vi "通信并与其他模块交互 (子VI).vi"() -> ()   [LabVIEW 2016, in "质控单元.lvlib"]
uses:
  <vilib>/Plasmionique/MB Master/MB_Master_TCP/MB_Master_TCP.lvclass
  D:/Program Files (x86)/National Instruments/LabVIEW 2016/vi.lib/Plasmionique/MB Master/MB_Master/MB_Master.lvclass
  <vilib>/Plasmionique/MB Master/MB_Master/MB_Master.lvclass
  <vilib>/Plasmionique/MB Master/MB Master.lvlib
  <vilib>/Utility/config.llb/NI_LVConfig.lvlib
panel:
  out "队列中元素数量":i32
  out "CODCr测量状态":u16[](array[numeric])
  out "CODMn测量状态":u16[](array[numeric])
  out "总氮测量状态":u16[](array[numeric])
  out "总磷测量状态":u16[](array[numeric])
  out "氨氮测量状态":u16[](array[numeric])
  out "通讯状态":bool
  in  "starting address 6":u16
  in  "values 6":u16[](array[numeric])
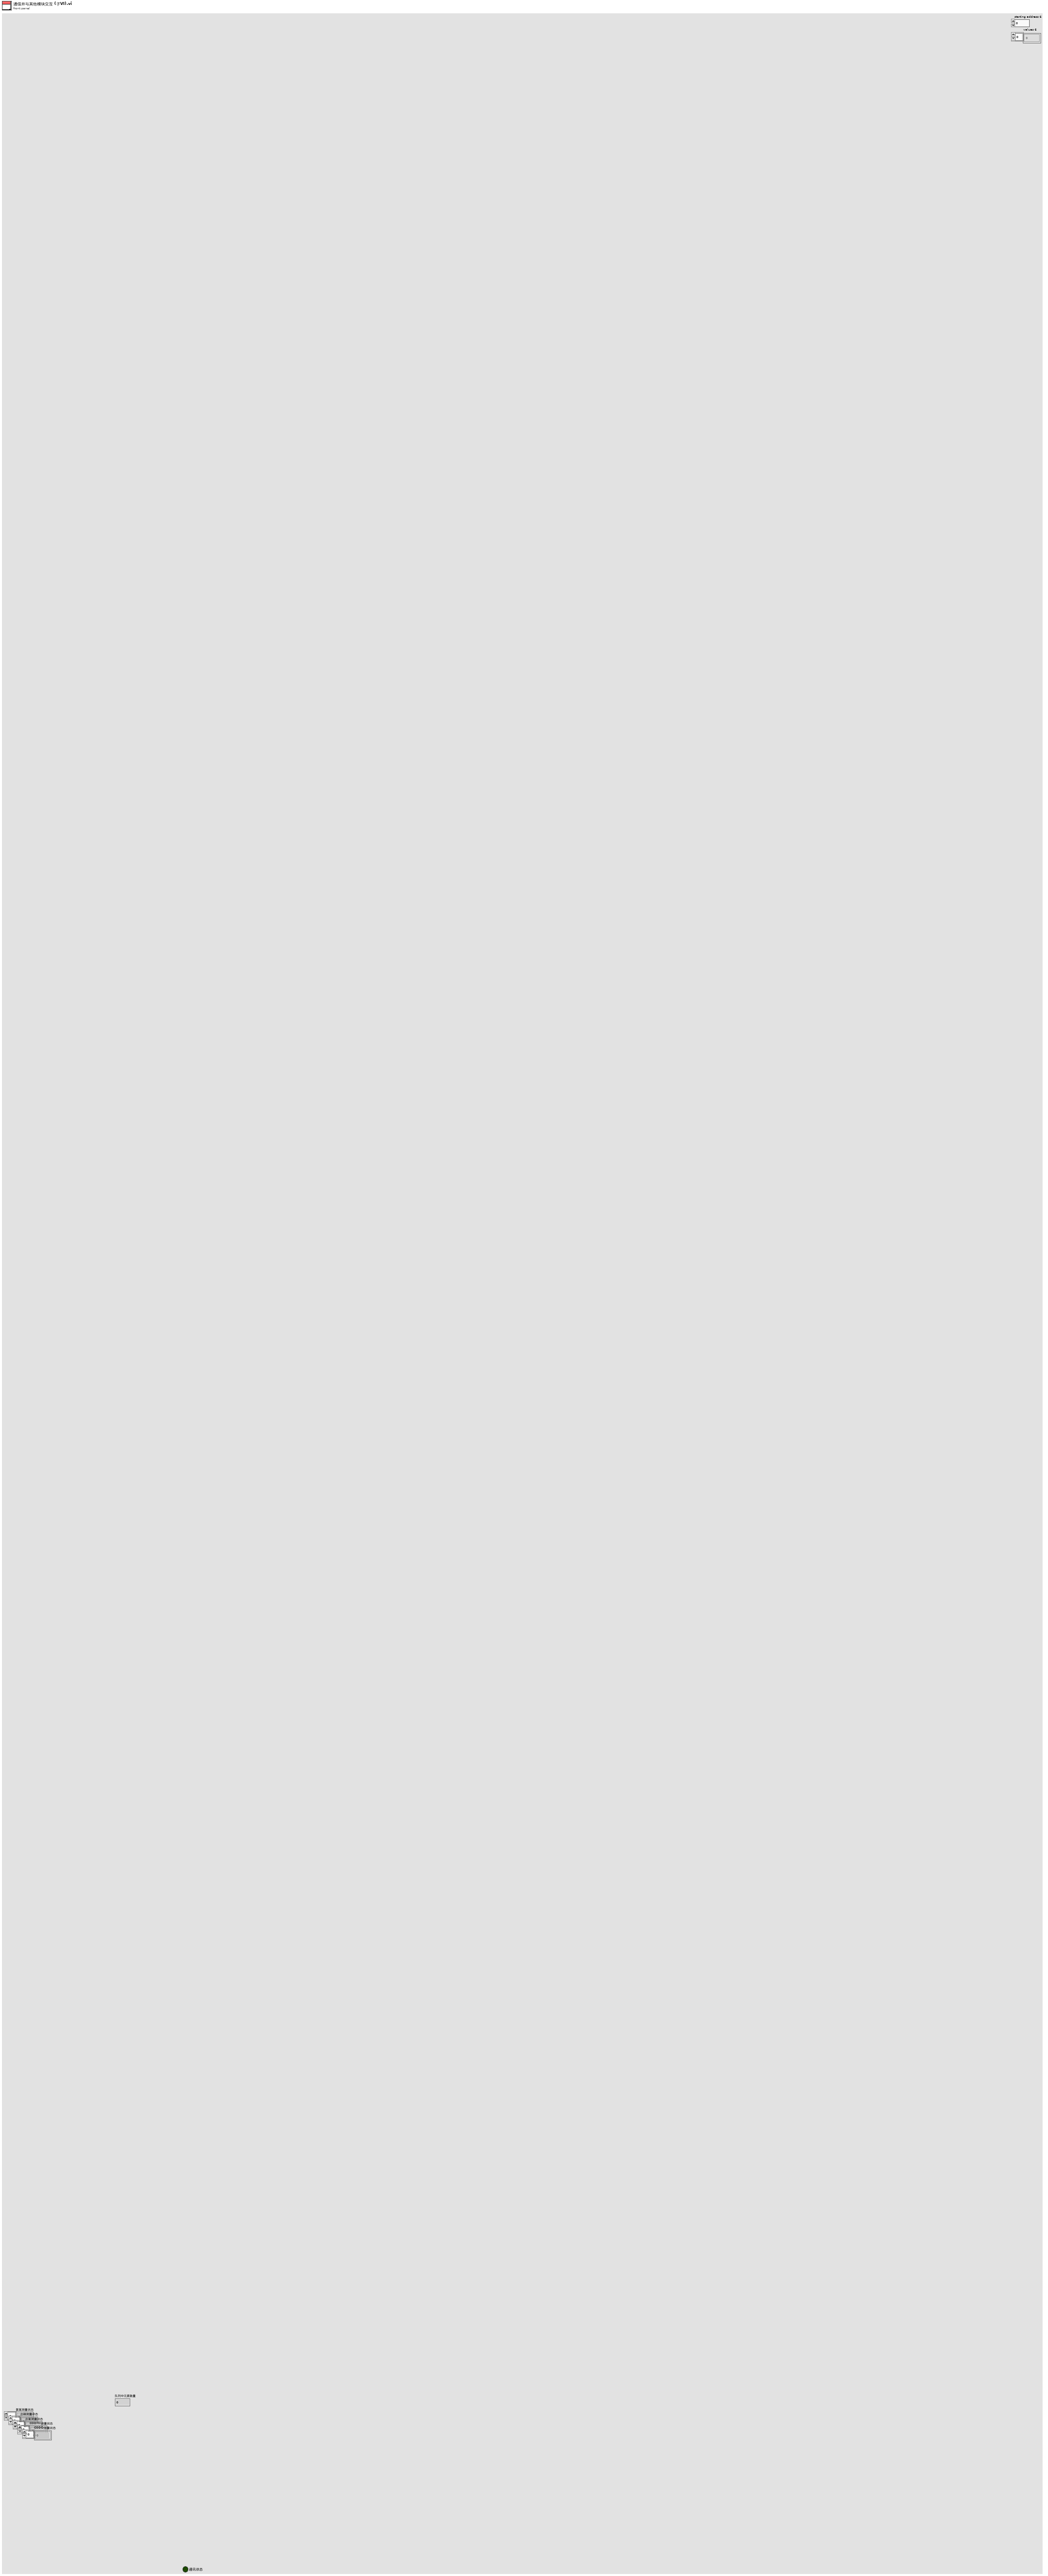
[diagram p1: front panel]
types:
  T1 = cluster{"仪器":enum16{"", "氨氮", "总磷", "总氮", "CODMn", "CODCr"}, "启动命令":enum16{"启动水样流程", "启动加标流程", "排液", "停止", "柱塞泵启动"}}
  T2 = cluster{"Registers[0]":u16, "Registers[1]":u16, "Registers[2]":u16, "Registers[3]":u16, "Registers[4]":u16, "Registers[5]":u16, "Registers[6]":u16, "Registers[7]":u16, "Registers[8]":u16, "Registers[9]":u16, "Registers[10]":u16, "Registers[11]":u16, "Registers[12]":u16, "Registers[13]":u16, "Registers[14]":u16, "Registers[15]":u16, "Registers[16]":u16, "Registers[17]":u16, "Registers[18]":u16, "Registers[19]":u16, "Registers[20]":u16, "Registers[21]":u16, "Registers[22]":u16, "Registers[23]":u16, "Registers[24]":u16, "Registers[25]":u16, "Registers[26]":u16, "Registers[27]":u16, "Registers[28]":u16, "Registers[29]":u16, "Registers[30]":u16, "Registers[31]":u16, "Registers[32]":u16, "Registers[33]":u16, "Registers[34]":u16, "Registers[35]":u16, "Registers[36]":u16, "Registers[37]":u16, "Registers[38]":u16, "Registers[39]":u16, "Registers[40]":u16, "Registers[41]":u16, "Registers[42]":u16, "Registers[43]":u16, "Registers[44]":u16, "Registers[45]":u16, "Registers[46]":u16, "Registers[47]":u16, "Registers[48]":u16, "Registers[49]":u16, "Registers[50]":u16, "Registers[51]":u16, "Registers[52]":u16, "Registers[53]":u16, "Registers[54]":u16, "Registers[55]":u16, "Registers[56]":u16}
  T3 = cluster{"因子编码":u32, "单位":u16, "标样参考值":sgl, "水样数据时间":timestamp, "水样实测值":sgl, "水样数据标识":string, "标样数据时间":timestamp, "标样实测值":sgl, "标样数据标识":string, "空白数据时间":timestamp, "空白实测值":sgl, "空白数据标识":string, "零点核查数据时间":timestamp, "零点核查实测值":sgl, "零点核查数据标识":string, "跨度核查数据时间":timestamp, "跨度核查实测值":sgl, "跨度核查数据标识":string, "加标回收数据时间":timestamp, "加标回收实测值":sgl, "加标回收数据标识":string, "平行样数据时间":timestamp, "平行样实测值":sgl, "平行样数据标识":string}
  T4 = cluster{"系统时间":timestamp, "工作状态":enum16{"空闲", "水样测试", "标样核查", "零点核查", "跨度核查", "空白测试", "平行样测试", "加标回收", "空白校准", "标样校准", "初始化（清洗）"}, "测量模式":enum16{"待机", "连续模式", "周期模式", "定点模式", "受控模式", "手动模式"}, "告警代码":enum16{"无告警", "缺试剂告警", "缺水样告警", "缺蒸馏水告警", "缺标液告警", "仪表漏液告警", "标定异常告警", "超量程告警", "加热异常", "低试剂预警", "超上限告警", "超下限告警", "仪表内部其他异常", "滴定异常告警", "电极异常告警", "量程切换告警", "参数设置告警", "PH电极电位异常", "电导率电极异常", "浊度光度异常", "溶解氧电极异常", "溶解氧光强异常", "温度异常告警", "PH异常告警", "溶解氧异常告警", "电导率异常告警", "浊度异常告警", "叶绿素异常告警", "藻密度异常告警", "蓝绿藻异常告警", "ORP异常告警", "氨氮异常告警", "清洁刷异常告警", "SD卡异常告警", "蓝牙异常告警", "Wifi异常告警", "流程异常告警"}, "故障代码":enum16{"无故障", "电机故障", "温度故障", "通讯故障", "滴定故障"}, "日志代码":u16, "软件版本":u16, "F0":sgl, "F1":sgl, "F2":sgl, "F3":sgl, "T":sgl, "H":sgl, "id":u16, "flowid":u16, "量程":u16, "总磷控温温度1":sgl, "营养盐控温温度2":sgl, "ADC":sgl}
  T5 = typedef "NI_LVConfig.lvlib/Config Data RefNum.ctl" = refnum<k1>
  T6 = cluster{"仪器":enum16{"", "氨氮", "总磷", "总氮", "CODMn", "CODCr"}, "starting address":u16, "value":u16}
  T7 = cluster{"starting address":u16, "values":u16[], "Slave ID":u8}
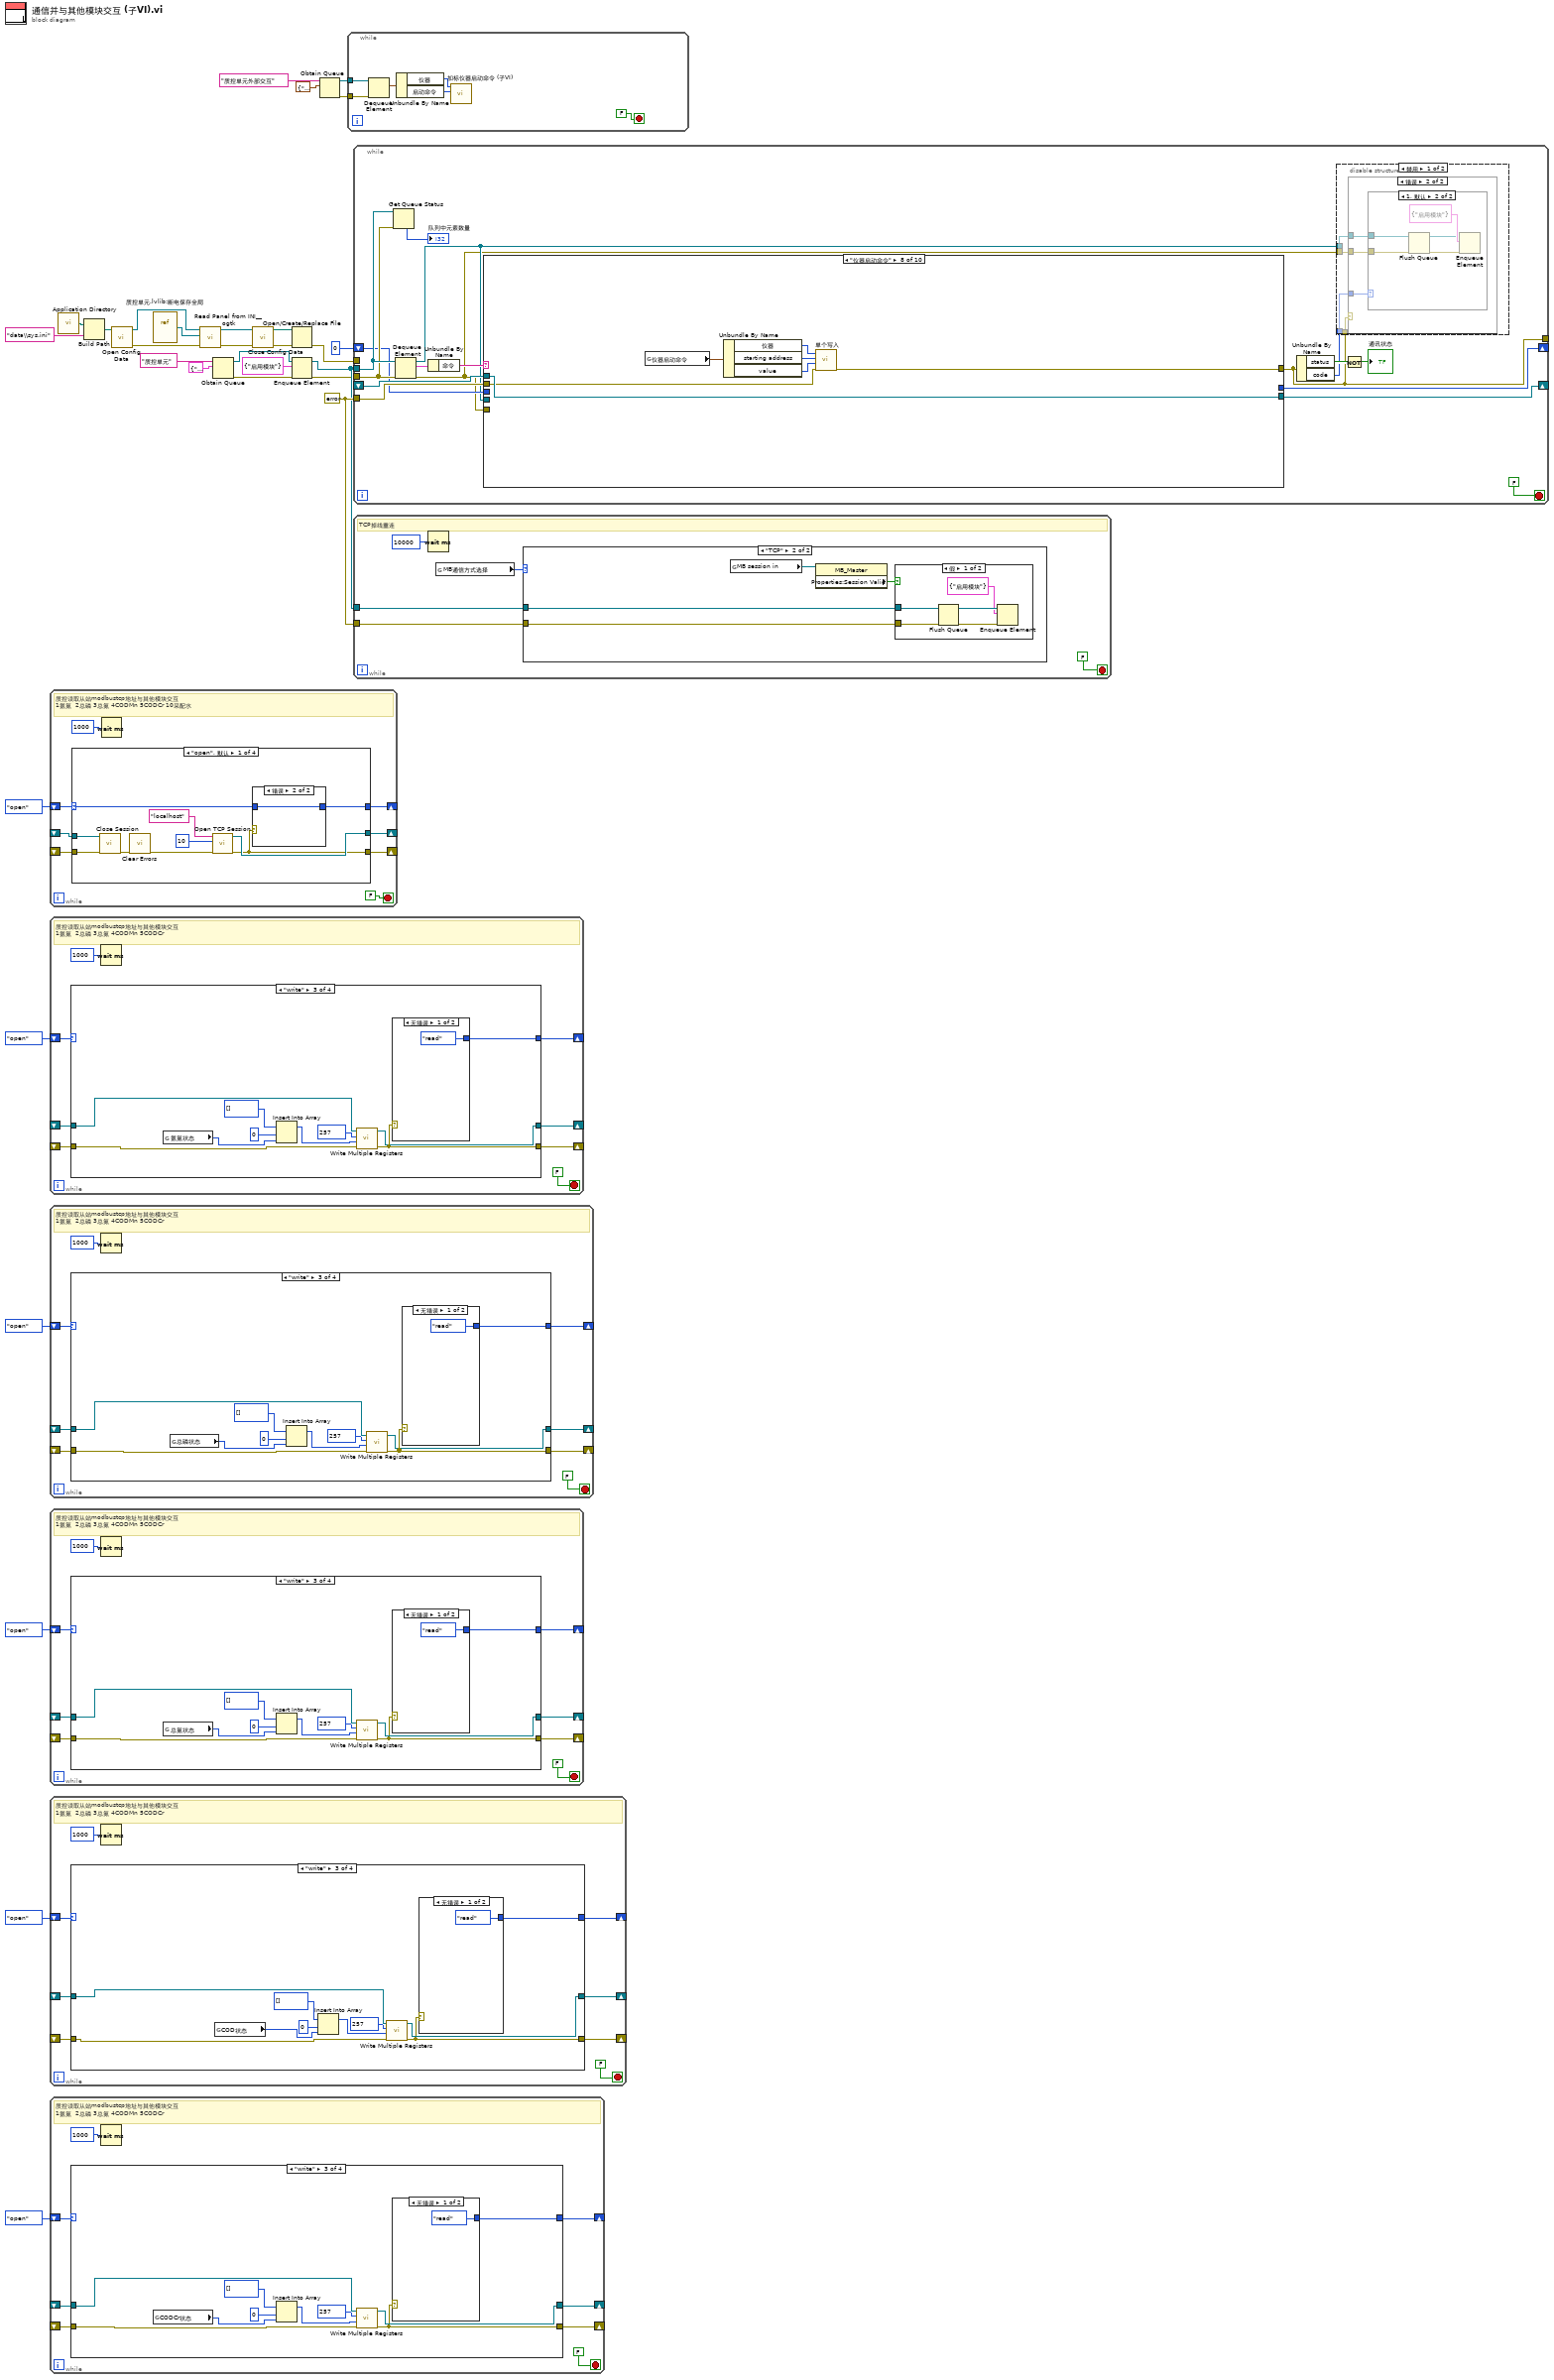
[diagram p0: block diagram]
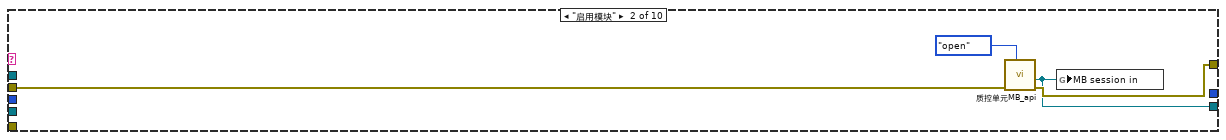
[diagram p8: hidden frame]
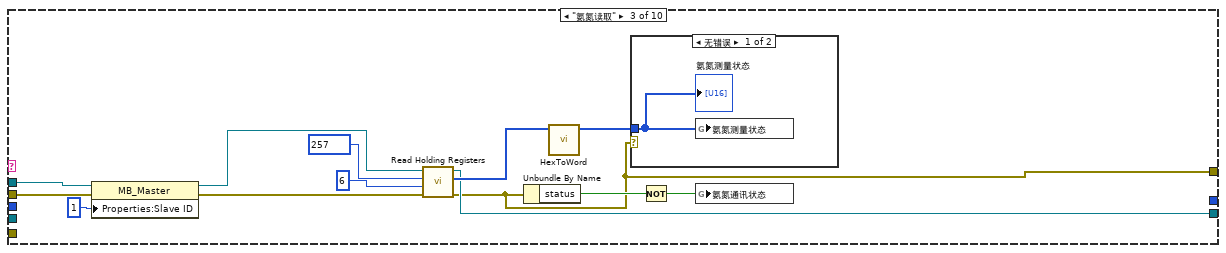
[diagram p9: hidden frame]
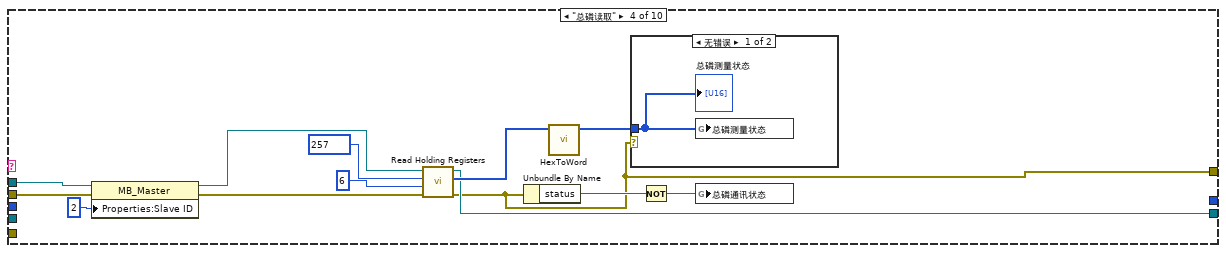
[diagram p11: hidden frame]
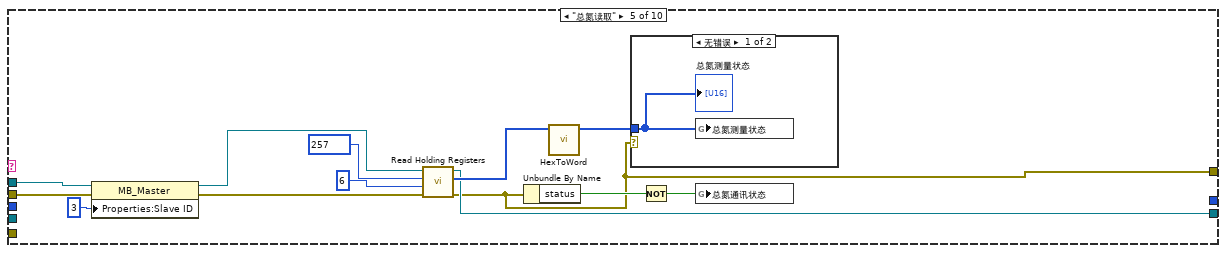
[diagram p13: hidden frame]
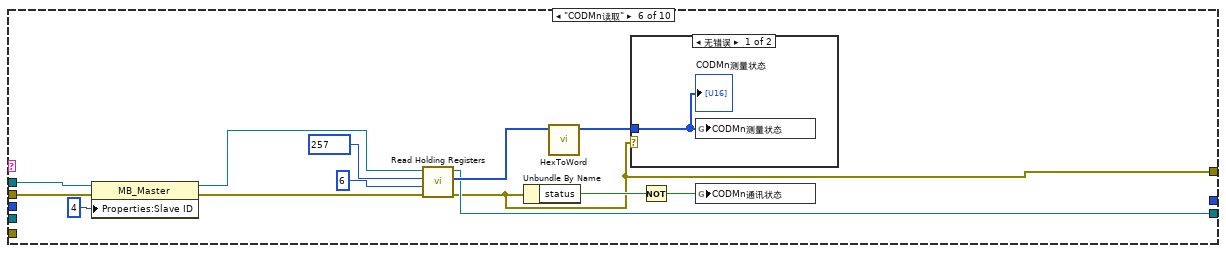
[diagram p15: hidden frame]
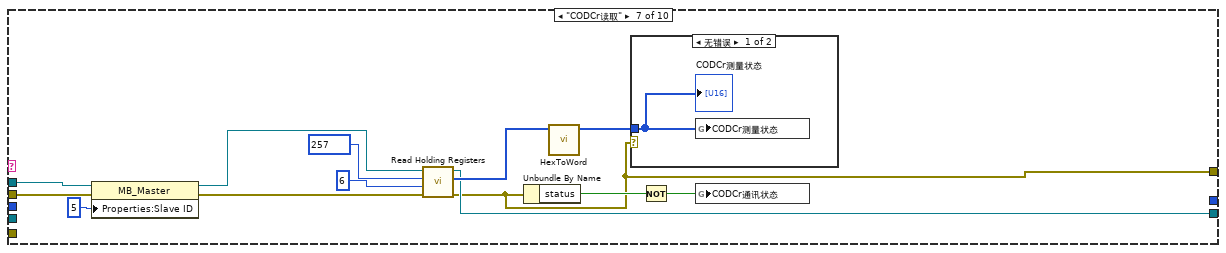
[diagram p17: hidden frame]
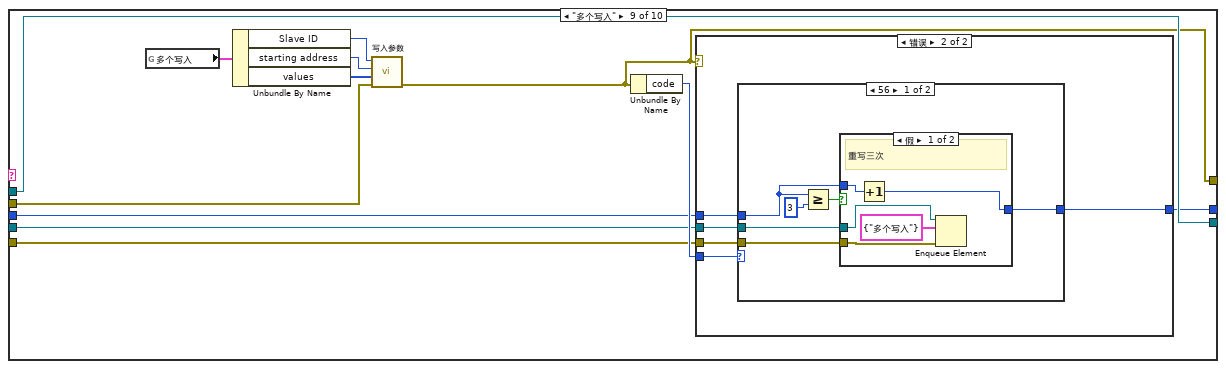
[diagram p19: hidden frame]
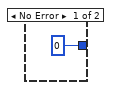
[diagram p20: hidden frame]
diagram:
  w8 = errorcluster {"status"=FALSE, "code"=0, "source"=""} ("error out")
  n1 = while {
    shift-right: [w36] -> _
    shift-left: _ -> [w38]
    shift-right: [w35] -> _
    shift-left: _ -> [w37]
    shift-right: [w32] -> _
    shift-left: enum16{"open", "read", "write", "close"}."open" -> [w33]
    stop <- FALSE stop-if-true
    # "质控读取从站modbustcp地址与其他模块交互\n1氨氮  2总磷 3总氮 4CODMn 5CODCr 10采配水"
    n2 = case shown="\"open\", 默认" w33 {
      selector: w33 -> [w40 _ _ _]
      tunnel: w38 -> [w45 w60 w68 w76]
      tunnel: w37 -> [w44 w57 w67 w75]
      tunnel: [w46 w53 w66 w76] -> w36
      tunnel: [w41 w52 w65 w73] -> w35
      tunnel: [w39 w56 w69 enum16{"open", "read", "write", "close"}."open"] -> w32
      frame "open", Default {
        n3 = call-dynamic "Close Session.vi"("error in (no error)"=w44, "MB session in"=w45) -> ("error out"=w43:errorcluster)  [unwired: 9 in]
        n4 = call <vilib>:"Clear Errors.vi"("error in (no error)"=w43) -> ("error out"=w42:errorcluster)  [unwired: 5 in, 1 out]
        n5 = call <vilib>:"Open TCP Session.vi"("error in (no error)"=w42, "Port (502)"=u16 10, "IP Address"="localhost") -> ("error out"=w41:errorcluster, "MB_TCP session"=w46:refnum<class "MB_Master_TCP.lvclass">)  [unwired: 7 in]
        n6 = case shown="错误" w41 {
          tunnel: w40 -> [w50 w51]
          tunnel: [w49 w51] -> w39
          frame No Error {
            n7 = Increment(x=w50) -> (x+1=w49:enum16{"open", "read", "write", "close"})
          }
          frame Error {
          }
        }
      }
      frame "read" {
        # "测量数据"
        n8 = call <vilib>:"Read Holding Registers.vi"("error in (no error)"=w57, "quantity"=u16 57, "starting address"=u16 0, "MB session in"=w60) -> ("error out"=w52:errorcluster, "Registers"=w55:u16[], "MB session out"=w53:refnum<class "MB_Master.lvclass">)  [unwired: 5 in]
        n9 = Array To Cluster(array=w55) -> (cluster=w54:T2)
        n10 = case shown="无错误" w52 {
          tunnel: [enum16{"open", "read", "write", "close"}."read" enum16{"open", "read", "write", "close"}."close"] -> w56
          frame No Error {
          }
          frame Error {
          }
        }
        n11 = global write "与采配水交互全局.vi" "状态"(w54) -> ()
      }
      frame "write" {
        n12 = call <vilib>:"Write Multiple Registers.vi"("error in (no error)"=w67, "values"="values 6", "starting address"="starting address 6", "MB session in"=w68) -> ("error out"=w65:errorcluster, "MB session out"=w66:refnum<class "MB_Master.lvclass">)  [unwired: 6 in]
        n13 = case shown="无错误" w65 {
          tunnel: [enum16{"open", "read", "write", "close"}."read" enum16{"open", "read", "write", "close"}."close"] -> w69
          frame No Error {
          }
          frame Error {
          }
        }
      }
      frame "close" {
        n14 = call-dynamic "Close Session.vi"("error in (no error)"=w75, "MB session in"=w76) -> ("error out"=w74:errorcluster)  [unwired: 9 in]
        n15 = call <vilib>:"Clear Errors.vi"("error in (no error)"=w74) -> ("error out"=w73:errorcluster)  [unwired: 5 in, 1 out]
      }
    }
    n16 = Wait (ms)(milliseconds to wait=u32 1000 ("等待时间（毫秒）")) -> ()  [unwired: 1 out]
  }
  n17 = while {
    shift-right: [w82] -> _
    shift-left: _ -> [w84]
    shift-right: [w81] -> _
    shift-left: _ -> [w83]
    shift-right: [w78] -> _
    shift-left: enum16{"open", "read", "write", "close"}."open" -> [w79]
    stop <- FALSE stop-if-true
    # "质控读取从站modbustcp地址与其他模块交互\n1氨氮  2总磷 3总氮 4CODMn 5CODCr"
    n18 = case shown="\"write\"" w79 {
      selector: w79 -> [w86 _ _ _]
      tunnel: w84 -> [w91 w112 w123 w131]
      tunnel: w83 -> [w90 w109 w122 w130]
      tunnel: [w92 w103 w121 w131] -> w82
      tunnel: [w87 w102 w120 w128] -> w81
      tunnel: [w85 w108 w124 enum16{"open", "read", "write", "close"}."open"] -> w78
      frame "open", Default {
        n19 = call-dynamic "Close Session.vi"("error in (no error)"=w90, "MB session in"=w91) -> ("error out"=w89:errorcluster)  [unwired: 9 in]
        n20 = call <vilib>:"Clear Errors.vi"("error in (no error)"=w89) -> ("error out"=w88:errorcluster)  [unwired: 5 in, 1 out]
        n21 = call <vilib>:"Open TCP Session.vi"("error in (no error)"=w88, "Port (502)"=u16 1, "IP Address"="localhost") -> ("error out"=w87:errorcluster, "MB_TCP session"=w92:refnum<class "MB_Master_TCP.lvclass">)  [unwired: 7 in]
        n22 = case shown="错误" w87 {
          tunnel: w86 -> [w96 w97]
          tunnel: [w95 w97] -> w85
          frame No Error {
            n23 = Increment(x=w96) -> (x+1=w95:enum16{"open", "read", "write", "close"})
          }
          frame Error {
          }
        }
      }
      frame "read" {
        # "状态告警"
        # "测量数据"
        n24 = call <vilib>:"Read Holding Registers.vi"("error in (no error)"=w109, "quantity"=u16 83, "starting address"=u16 4096, "MB session in"=w112) -> ("error out"=w104:errorcluster, "Registers"=w101:u16[], "MB session out"=w105:refnum<class "MB_Master.lvclass">)  [unwired: 5 in]
        n25 = call "交互测量数据区解析.vi"("数组"=w101) -> ("测量数据区"=w100:T3)  [unwired: 10 in]
        n26 = call <vilib>:"Read Holding Registers.vi"("error in (no error)"=w104, "quantity"=u16 24, "starting address"=u16 4224, "MB session in"=w105) -> ("error out"=w102:errorcluster, "Registers"=w99:u16[], "MB session out"=w103:refnum<class "MB_Master.lvclass">)  [unwired: 5 in]
        n27 = case shown="无错误" w102 {
          tunnel: [enum16{"open", "read", "write", "close"}."write" enum16{"open", "read", "write", "close"}."close"] -> w108
          frame No Error {
          }
          frame Error {
          }
        }
        n28 = call "交互状态告警区解析.vi"("数组"=w99) -> ("状态告警区"=w98:T4)  [unwired: 10 in]
        n29 = global write "与氨氮交互全局.vi" "氨氮测量数据区"(w100) -> ()
        n30 = global write "与氨氮交互全局.vi" "氨氮状态告警区"(w98) -> ()
      }
      frame "write" {
        n31 = global read "加标回收状态全局变量.vi" "氨氮状态"() -> (w118:u16)
        n32 = Insert Into Array(array=u16[] [] ("values 6"), index=0 ("索引"), new element=w118) -> (w115:u16[])
        n33 = call <vilib>:"Write Multiple Registers.vi"("error in (no error)"=w122, "values"=w115, "starting address"=u16 257, "MB session in"=w123) -> ("error out"=w120:errorcluster, "MB session out"=w121:refnum<class "MB_Master.lvclass">)  [unwired: 6 in]
        n34 = case shown="无错误" w120 {
          tunnel: [enum16{"open", "read", "write", "close"}."read" enum16{"open", "read", "write", "close"}."close"] -> w124
          frame No Error {
          }
          frame Error {
          }
        }
      }
      frame "close" {
        n35 = call-dynamic "Close Session.vi"("error in (no error)"=w130, "MB session in"=w131) -> ("error out"=w129:errorcluster)  [unwired: 9 in]
        n36 = call <vilib>:"Clear Errors.vi"("error in (no error)"=w129) -> ("error out"=w128:errorcluster)  [unwired: 5 in, 1 out]
      }
    }
    n37 = Wait (ms)(milliseconds to wait=u32 1000 ("等待时间（毫秒）")) -> ()  [unwired: 1 out]
  }
  n38 = while {
    shift-right: [w137] -> _
    shift-left: _ -> [w139]
    shift-right: [w136] -> _
    shift-left: _ -> [w138]
    shift-right: [w133] -> _
    shift-left: enum16{"open", "read", "write", "close"}."open" -> [w134]
    stop <- FALSE stop-if-true
    # "质控读取从站modbustcp地址与其他模块交互\n1氨氮  2总磷 3总氮 4CODMn 5CODCr"
    n39 = case shown="\"write\"" w134 {
      selector: w134 -> [w141 _ _ _]
      tunnel: w139 -> [w146 w167 w178 w186]
      tunnel: w138 -> [w145 w164 w177 w185]
      tunnel: [w147 w158 w176 w186] -> w137
      tunnel: [w142 w157 w175 w183] -> w136
      tunnel: [w140 w163 w179 enum16{"open", "read", "write", "close"}."open"] -> w133
      frame "open", Default {
        n40 = call-dynamic "Close Session.vi"("error in (no error)"=w145, "MB session in"=w146) -> ("error out"=w144:errorcluster)  [unwired: 9 in]
        n41 = call <vilib>:"Clear Errors.vi"("error in (no error)"=w144) -> ("error out"=w143:errorcluster)  [unwired: 5 in, 1 out]
        n42 = call <vilib>:"Open TCP Session.vi"("error in (no error)"=w143, "Port (502)"=u16 2, "IP Address"="localhost") -> ("error out"=w142:errorcluster, "MB_TCP session"=w147:refnum<class "MB_Master_TCP.lvclass">)  [unwired: 7 in]
        n43 = case shown="无错误" w142 {
          tunnel: w141 -> [w151 w152]
          tunnel: [w150 w152] -> w140
          frame No Error {
            n44 = Increment(x=w151) -> (x+1=w150:enum16{"open", "read", "write", "close"})
          }
          frame Error {
          }
        }
      }
      frame "read" {
        # "状态告警"
        # "测量数据"
        n45 = call <vilib>:"Read Holding Registers.vi"("error in (no error)"=w164, "quantity"=u16 83, "starting address"=u16 4096, "MB session in"=w167) -> ("error out"=w159:errorcluster, "Registers"=w156:u16[], "MB session out"=w160:refnum<class "MB_Master.lvclass">)  [unwired: 5 in]
        n46 = call "交互测量数据区解析.vi"("数组"=w156) -> ("测量数据区"=w154:T3)  [unwired: 10 in]
        n47 = call <vilib>:"Read Holding Registers.vi"("error in (no error)"=w159, "quantity"=u16 24, "starting address"=u16 4224, "MB session in"=w160) -> ("error out"=w157:errorcluster, "Registers"=w155:u16[], "MB session out"=w158:refnum<class "MB_Master.lvclass">)  [unwired: 5 in]
        n48 = case shown="无错误" w157 {
          tunnel: [enum16{"open", "read", "write", "close"}."write" enum16{"open", "read", "write", "close"}."close"] -> w163
          frame No Error {
          }
          frame Error {
          }
        }
        n49 = call "交互状态告警区解析.vi"("数组"=w155) -> ("状态告警区"=w153:T4)  [unwired: 10 in]
        n50 = global write "与总磷交互全局.vi" "总磷测量数据区"(w154) -> ()
        n51 = global write "与总磷交互全局.vi" "总磷状态告警区"(w153) -> ()
      }
      frame "write" {
        n52 = global read "加标回收状态全局变量.vi" "总磷状态"() -> (w173:u16)
        n53 = Insert Into Array(array=u16[] [] ("values 6"), index=0 ("索引"), new element=w173) -> (w170:u16[])
        n54 = call <vilib>:"Write Multiple Registers.vi"("error in (no error)"=w177, "values"=w170, "starting address"=u16 257, "MB session in"=w178) -> ("error out"=w175:errorcluster, "MB session out"=w176:refnum<class "MB_Master.lvclass">)  [unwired: 6 in]
        n55 = case shown="无错误" w175 {
          tunnel: [enum16{"open", "read", "write", "close"}."read" enum16{"open", "read", "write", "close"}."close"] -> w179
          frame No Error {
          }
          frame Error {
          }
        }
      }
      frame "close" {
        n56 = call-dynamic "Close Session.vi"("error in (no error)"=w185, "MB session in"=w186) -> ("error out"=w184:errorcluster)  [unwired: 9 in]
        n57 = call <vilib>:"Clear Errors.vi"("error in (no error)"=w184) -> ("error out"=w183:errorcluster)  [unwired: 5 in, 1 out]
      }
    }
    n58 = Wait (ms)(milliseconds to wait=u32 1000 ("等待时间（毫秒）")) -> ()  [unwired: 1 out]
  }
  n59 = while {
    shift-right: [w192] -> _
    shift-left: _ -> [w194]
    shift-right: [w191] -> _
    shift-left: _ -> [w193]
    shift-right: [w188] -> _
    shift-left: enum16{"open", "read", "write", "close"}."open" -> [w189]
    stop <- FALSE stop-if-true
    # "质控读取从站modbustcp地址与其他模块交互\n1氨氮  2总磷 3总氮 4CODMn 5CODCr"
    n60 = case shown="\"write\"" w189 {
      selector: w189 -> [w196 _ _ _]
      tunnel: w194 -> [w201 w222 w233 w241]
      tunnel: w193 -> [w200 w219 w232 w240]
      tunnel: [w202 w213 w231 w241] -> w192
      tunnel: [w197 w212 w230 w238] -> w191
      tunnel: [w195 w218 w234 enum16{"open", "read", "write", "close"}."open"] -> w188
      frame "open", Default {
        n61 = call-dynamic "Close Session.vi"("error in (no error)"=w200, "MB session in"=w201) -> ("error out"=w199:errorcluster)  [unwired: 9 in]
        n62 = call <vilib>:"Clear Errors.vi"("error in (no error)"=w199) -> ("error out"=w198:errorcluster)  [unwired: 5 in, 1 out]
        n63 = call <vilib>:"Open TCP Session.vi"("error in (no error)"=w198, "Port (502)"=u16 3, "IP Address"="localhost") -> ("error out"=w197:errorcluster, "MB_TCP session"=w202:refnum<class "MB_Master_TCP.lvclass">)  [unwired: 7 in]
        n64 = case shown="无错误" w197 {
          tunnel: w196 -> [w206 w207]
          tunnel: [w205 w207] -> w195
          frame No Error {
            n65 = Increment(x=w206) -> (x+1=w205:enum16{"open", "read", "write", "close"})
          }
          frame Error {
          }
        }
      }
      frame "read" {
        # "状态告警"
        # "测量数据"
        n66 = call <vilib>:"Read Holding Registers.vi"("error in (no error)"=w219, "quantity"=u16 83, "starting address"=u16 4096, "MB session in"=w222) -> ("error out"=w214:errorcluster, "Registers"=w211:u16[], "MB session out"=w215:refnum<class "MB_Master.lvclass">)  [unwired: 5 in]
        n67 = call "交互测量数据区解析.vi"("数组"=w211) -> ("测量数据区"=w209:T3)  [unwired: 10 in]
        n68 = call <vilib>:"Read Holding Registers.vi"("error in (no error)"=w214, "quantity"=u16 24, "starting address"=u16 4224, "MB session in"=w215) -> ("error out"=w212:errorcluster, "Registers"=w210:u16[], "MB session out"=w213:refnum<class "MB_Master.lvclass">)  [unwired: 5 in]
        n69 = case shown="无错误" w212 {
          tunnel: [enum16{"open", "read", "write", "close"}."write" enum16{"open", "read", "write", "close"}."close"] -> w218
          frame No Error {
          }
          frame Error {
          }
        }
        n70 = call "交互状态告警区解析.vi"("数组"=w210) -> ("状态告警区"=w208:T4)  [unwired: 10 in]
        n71 = global write "与总氮交互全局.vi" "总氮测量数据区"(w209) -> ()
        n72 = global write "与总氮交互全局.vi" "总氮状态告警区"(w208) -> ()
      }
      frame "write" {
        n73 = global read "加标回收状态全局变量.vi" "总氮状态"() -> (w228:u16)
        n74 = Insert Into Array(array=u16[] [] ("values 6"), index=0 ("索引"), new element=w228) -> (w226:u16[])
        n75 = call <vilib>:"Write Multiple Registers.vi"("error in (no error)"=w232, "values"=w226, "starting address"=u16 257, "MB session in"=w233) -> ("error out"=w230:errorcluster, "MB session out"=w231:refnum<class "MB_Master.lvclass">)  [unwired: 6 in]
        n76 = case shown="无错误" w230 {
          tunnel: [enum16{"open", "read", "write", "close"}."read" enum16{"open", "read", "write", "close"}."close"] -> w234
          frame No Error {
          }
          frame Error {
          }
        }
      }
      frame "close" {
        n77 = call-dynamic "Close Session.vi"("error in (no error)"=w240, "MB session in"=w241) -> ("error out"=w239:errorcluster)  [unwired: 9 in]
        n78 = call <vilib>:"Clear Errors.vi"("error in (no error)"=w239) -> ("error out"=w238:errorcluster)  [unwired: 5 in, 1 out]
      }
    }
    n79 = Wait (ms)(milliseconds to wait=u32 1000 ("等待时间（毫秒）")) -> ()  [unwired: 1 out]
  }
  n80 = while {
    shift-right: [w247] -> _
    shift-left: _ -> [w249]
    shift-right: [w246] -> _
    shift-left: _ -> [w248]
    shift-right: [w243] -> _
    shift-left: enum16{"open", "read", "write", "close"}."open" -> [w244]
    stop <- FALSE stop-if-true
    # "质控读取从站modbustcp地址与其他模块交互\n1氨氮  2总磷 3总氮 4CODMn 5CODCr"
    n81 = case shown="\"write\"" w244 {
      selector: w244 -> [w251 _ _ _]
      tunnel: w249 -> [w256 w287 w298 w306]
      tunnel: w248 -> [w255 w284 w297 w305]
      tunnel: [w257 w282 w296 w306] -> w247
      tunnel: [w252 w281 w295 w303] -> w246
      tunnel: [w250 w283 w299 enum16{"open", "read", "write", "close"}."open"] -> w243
      frame "open", Default {
        n82 = call-dynamic "Close Session.vi"("error in (no error)"=w255, "MB session in"=w256) -> ("error out"=w254:errorcluster)  [unwired: 9 in]
        n83 = call <vilib>:"Clear Errors.vi"("error in (no error)"=w254) -> ("error out"=w253:errorcluster)  [unwired: 5 in, 1 out]
        n84 = call <vilib>:"Open TCP Session.vi"("error in (no error)"=w253, "Port (502)"=u16 4, "IP Address"="localhost") -> ("error out"=w252:errorcluster, "MB_TCP session"=w257:refnum<class "MB_Master_TCP.lvclass">)  [unwired: 7 in]
        n85 = case shown="无错误" w252 {
          tunnel: w251 -> [w261 w262]
          tunnel: [w260 w262] -> w250
          frame No Error {
            n86 = Increment(x=w261) -> (x+1=w260:enum16{"open", "read", "write", "close"})
          }
          frame Error {
          }
        }
      }
      frame "read" {
        # "测量数据"
        n87 = call <vilib>:"Read Holding Registers.vi"("error in (no error)"=w284, "quantity"=u16 30, "starting address"=u16 0, "MB session in"=w287) -> ("error out"=w281:errorcluster, "Registers"=w280:u16[], "MB session out"=w282:refnum<class "MB_Master.lvclass">)  [unwired: 5 in]
        n88 = case shown="无错误" w281 {
          tunnel: [enum16{"open", "read", "write", "close"}."write" enum16{"open", "read", "write", "close"}."close"] -> w283
          frame No Error {
          }
          frame Error {
          }
        }
        n89 = Index Array(array=w280) -> (element #1=w279:u16, element #2=w278:u16, element #3=w277:u16, element #4=w273:u16, element #5=w272:u16, element #6=w271:u16, element #7=w270:u16, element #8=w268:u16, element #9=w267:u16, element #10=w266:u16)  [unwired: 10 in]
        n90 = global write "与CODMn交互全局.vi" "CODMn工作状态"(w279) -> ()
        n91 = global write "与CODMn交互全局.vi" "多列列表框"(w273) -> ()
        n92 = Build Array(w272, w271, w270, w268, w267, w266) -> (w269:u16[])
        n93 = Build Array(w278, w277) -> (w276:u16[])
        n94 = call "HexToCDABFloat.vi"("数组"=w276) -> ("FLOAT"=w275:sgl[])  [unwired: 10 in]
        n95 = call "HexToDate.vi"("数组"=w269) -> ("DATE"=w265:timestamp[])  [unwired: 10 in]
        n96 = Index Array(array=w265) -> (element #1=w264:timestamp, element #2=w263:timestamp)  [unwired: 2 in]
        n97 = global write "与CODMn交互全局.vi" "加标回收启动时间"(w264) -> ()
        n98 = global write "与CODMn交互全局.vi" "水样启动时间"(w263) -> ()
        n99 = Index Array(array=w275) -> (element=w274:sgl)  [unwired: 1 in]
        n100 = global write "与CODMn交互全局.vi" "COD浓度（mg/L)"(w274) -> ()
      }
      frame "write" {
        n101 = global read "加标回收状态全局变量.vi" "COD状态"() -> (w293:u16)
        n102 = Insert Into Array(array=u16[] [] ("values 6"), index=0 ("索引"), new element=w293) -> (w291:u16[])
        n103 = call <vilib>:"Write Multiple Registers.vi"("error in (no error)"=w297, "values"=w291, "starting address"=u16 257, "MB session in"=w298) -> ("error out"=w295:errorcluster, "MB session out"=w296:refnum<class "MB_Master.lvclass">)  [unwired: 6 in]
        n104 = case shown="无错误" w295 {
          tunnel: [enum16{"open", "read", "write", "close"}."read" enum16{"open", "read", "write", "close"}."close"] -> w299
          frame No Error {
          }
          frame Error {
          }
        }
      }
      frame "close" {
        n105 = call-dynamic "Close Session.vi"("error in (no error)"=w305, "MB session in"=w306) -> ("error out"=w304:errorcluster)  [unwired: 9 in]
        n106 = call <vilib>:"Clear Errors.vi"("error in (no error)"=w304) -> ("error out"=w303:errorcluster)  [unwired: 5 in, 1 out]
      }
    }
    n107 = Wait (ms)(milliseconds to wait=u32 1000 ("等待时间（毫秒）")) -> ()  [unwired: 1 out]
  }
  n108 = while {
    shift-right: [w312] -> _
    shift-left: _ -> [w314]
    shift-right: [w311] -> _
    shift-left: _ -> [w313]
    shift-right: [w308] -> _
    shift-left: enum16{"open", "read", "write", "close"}."open" -> [w309]
    stop <- FALSE stop-if-true
    # "质控读取从站modbustcp地址与其他模块交互\n1氨氮  2总磷 3总氮 4CODMn 5CODCr"
    n109 = case shown="\"write\"" w309 {
      selector: w309 -> [w316 _ _ _]
      tunnel: w314 -> [w321 w342 w353 w361]
      tunnel: w313 -> [w320 w339 w352 w360]
      tunnel: [w322 w333 w351 w361] -> w312
      tunnel: [w317 w332 w350 w358] -> w311
      tunnel: [w315 w338 w354 enum16{"open", "read", "write", "close"}."open"] -> w308
      frame "open", Default {
        n110 = call-dynamic "Close Session.vi"("error in (no error)"=w320, "MB session in"=w321) -> ("error out"=w319:errorcluster)  [unwired: 9 in]
        n111 = call <vilib>:"Clear Errors.vi"("error in (no error)"=w319) -> ("error out"=w318:errorcluster)  [unwired: 5 in, 1 out]
        n112 = call <vilib>:"Open TCP Session.vi"("error in (no error)"=w318, "Port (502)"=u16 5, "IP Address"="localhost") -> ("error out"=w317:errorcluster, "MB_TCP session"=w322:refnum<class "MB_Master_TCP.lvclass">)  [unwired: 7 in]
        n113 = case shown="无错误" w317 {
          tunnel: w316 -> [w326 w327]
          tunnel: [w325 w327] -> w315
          frame No Error {
            n114 = Increment(x=w326) -> (x+1=w325:enum16{"open", "read", "write", "close"})
          }
          frame Error {
          }
        }
      }
      frame "read" {
        # "状态告警"
        # "测量数据"
        n115 = call <vilib>:"Read Holding Registers.vi"("error in (no error)"=w339, "quantity"=u16 83, "starting address"=u16 4096, "MB session in"=w342) -> ("error out"=w334:errorcluster, "Registers"=w331:u16[], "MB session out"=w335:refnum<class "MB_Master.lvclass">)  [unwired: 5 in]
        n116 = call "交互测量数据区解析.vi"("数组"=w331) -> ("测量数据区"=w329:T3)  [unwired: 10 in]
        n117 = call <vilib>:"Read Holding Registers.vi"("error in (no error)"=w334, "quantity"=u16 24, "starting address"=u16 4224, "MB session in"=w335) -> ("error out"=w332:errorcluster, "Registers"=w330:u16[], "MB session out"=w333:refnum<class "MB_Master.lvclass">)  [unwired: 5 in]
        n118 = case shown="无错误" w332 {
          tunnel: [enum16{"open", "read", "write", "close"}."write" enum16{"open", "read", "write", "close"}."close"] -> w338
          frame No Error {
          }
          frame Error {
          }
        }
        n119 = call "交互状态告警区解析.vi"("数组"=w330) -> ("状态告警区"=w328:T4)  [unwired: 10 in]
        n120 = global write "与CODCr交互全局.vi" "CODCr测量数据区"(w329) -> ()
        n121 = global write "与CODCr交互全局.vi" "CODCr状态告警区"(w328) -> ()
      }
      frame "write" {
        n122 = global read "加标回收状态全局变量.vi" "CODCr状态"() -> (w348:u16)
        n123 = Insert Into Array(array=u16[] [] ("values 6"), index=0 ("索引"), new element=w348) -> (w346:u16[])
        n124 = call <vilib>:"Write Multiple Registers.vi"("error in (no error)"=w352, "values"=w346, "starting address"=u16 257, "MB session in"=w353) -> ("error out"=w350:errorcluster, "MB session out"=w351:refnum<class "MB_Master.lvclass">)  [unwired: 6 in]
        n125 = case shown="无错误" w350 {
          tunnel: [enum16{"open", "read", "write", "close"}."read" enum16{"open", "read", "write", "close"}."close"] -> w354
          frame No Error {
          }
          frame Error {
          }
        }
      }
      frame "close" {
        n126 = call-dynamic "Close Session.vi"("error in (no error)"=w360, "MB session in"=w361) -> ("error out"=w359:errorcluster)  [unwired: 9 in]
        n127 = call <vilib>:"Clear Errors.vi"("error in (no error)"=w359) -> ("error out"=w358:errorcluster)  [unwired: 5 in, 1 out]
      }
    }
    n128 = Wait (ms)(milliseconds to wait=u32 1000 ("等待时间（毫秒）")) -> ()  [unwired: 1 out]
  }
  n129 = call <vilib>:"Application Directory.vi"() -> ("Application Directory"=w19:path)
  n130 = Build Path(base path=w19, name or relative path="data\\sys.ini" ("名称或相对路径")) -> (appended path=w17:path)
  n131 = call <vilib>:"Open Config Data.vi"("configuration file path"=w17) -> ("error out"=w13:errorcluster, "refnum"=w16:T5)  [unwired: 8 in, 1 out]
  n132 = vi-ref "质控单元.lvlib:断电保存全局.vi"() -> (w15:refnum<vi>)
  n133 = call <userlib>:"Read Panel from INI__ogtk.vi"("error in (no error)"=w13, "VI ref"=w15, "refnum"=w16) -> ("error out"=w12:errorcluster, "refnum out"=w14:T5)  [unwired: 7 in]
  n134 = Obtain Queue(name (unnamed)="质控单元" ("名称（未命名）"), element data type=cluster{"命令":string} {"命令"="启用模块"} ("元素")) -> (queue out=w22:refnum<queue>, error out=w21:errorcluster)  [unwired: 3 in, 1 out]
  n135 = call <vilib>:"Close Config Data.vi"("error in (no error)"=w12, "refnum"=w14) -> ("error out"=w11:errorcluster, "file path"=w10:path)  [unwired: 8 in]
  n136 = Open/Create/Replace File(file path (use dialog)=w10, error in=w11) -> (error out=w9:errorcluster)  [unwired: 4 in, 2 out]
  n137 = Enqueue Element(queue=w22, element=cluster{"命令":string} {"命令"="启用模块"} ("元素"), error in (no error)=w21) -> (queue out=w3:refnum<queue>, error out=w2:errorcluster)  [unwired: 1 in, 1 out]
  n138 = Obtain Queue(name (unnamed)="质控单元外部交互" ("名称（未命名）"), element data type=T1 {"仪器"=enum."氨氮", "启动命令"=enum."启动水样流程"} ("元素")) -> (queue out=w5:refnum<queue>, error out=w4:errorcluster)  [unwired: 3 in, 1 out]
  n139 = while {
    tunnel: w5 -> [w367]
    tunnel: w4 -> [w366]
    stop <- FALSE stop-if-true
    n140 = Dequeue Element(queue=w367, error in (no error)=w366) -> (element=w365:T1)  [unwired: 1 in, 3 out]
    n141 = Unbundle By Name(w365) -> ("仪器"=w364:enum16{"", "氨氮", "总磷", "总氮", "CODMn", "CODCr"}, "启动命令"=w363:enum16{"启动水样流程", "启动加标流程", "排液", "停止", "柱塞泵启动"})
    n142 = call "加标仪器启动命令 (子VI).vi"("启动命令"=w363, "仪器"=w364) -> ()  [unwired: 9 in, 1 out]
  }
  n143 = while {
    tunnel: w3 -> [w375]
    tunnel: w2 -> [w374]
    shift-right: [w380] -> _
    shift-left: _ -> [w379]
    tunnel: w9 -> [_]
    tunnel: w8 -> [w377]
    tunnel: [w376] -> _
    shift-right: [w370] -> _
    shift-left: 0 -> [w371]
    stop <- FALSE stop-if-true
    n144 = Get Queue Status(queue=w375, error in (no error)=w374) -> (# elements in queue=→"队列中元素数量":i32)  [unwired: 1 in, 7 out]
    n145 = Dequeue Element(queue=w375, error in (no error)=w374) -> (queue out=w369:refnum<queue>, element=w384:cluster{"命令":string}, error out=w368:errorcluster)  [unwired: 1 in, 1 out]
    n146 = Unbundle By Name(w384) -> ("命令"=w383:string)
    n147 = case shown="\"仪器启动命令\"" w383 {
      tunnel: [w398 w399 w404 w418 w432 w446 w460 w478 w490 w511] -> w380
      tunnel: [w397 w402 w403 w417 w431 w445 w459 w479 w480 w512] -> w376
      tunnel: w379 -> [w398 _ w406 w420 w434 w448 w462 w478 w490 _]
      tunnel: w377 -> [w397 w400 w405 w419 w433 w447 w461 w477 w486 w513]
      tunnel: w371 -> [_ _ _ _ _ _ _ _ w484 _]
      tunnel: [_ _ _ _ _ _ _ _ w483 _] -> w370
      tunnel: w369 -> [_ _ _ _ _ _ _ _ w482 _]
      tunnel: w368 -> [_ _ _ _ _ _ _ _ w481 _]
      frame Default {
      }
      frame "启用模块" {
        n148 = call "质控单元MB_api.vi"("STEP"=enum16{"open", "read", "write", "close"}."open", "Error in"=w400) -> ("error out"=w402:errorcluster, "MB session out"=w399:refnum<class "MB_Master.lvclass">)  [unwired: 7 in, 1 out]
        n149 = global write "断电保存全局.vi" "MB session in"(w399) -> ()
      }
      frame "氨氮读取" {
        n150 = property class="MB_Master"(reference=w406, error in=w405, "Properties:Slave ID"=u8 1 ("Slave ID")) -> (reference out=w409:refnum<class "MB_Master.lvclass">, error out=w415:errorcluster)
        n151 = call <vilib>:"Read Holding Registers.vi"("error in (no error)"=w415, "quantity"=u16 6 ("number of holding registers"), "starting address"=u16 257, "MB session in"=w409) -> ("error out"=w403:errorcluster, "Registers"=w413:u16[], "MB session out"=w404:refnum<class "MB_Master.lvclass">)  [unwired: 5 in]
        n152 = Unbundle By Name(w403) -> ("status"=w408:bool)
        n153 = call "HexToWord.vi"("数组"=w413) -> ("WORD"=w414:u16[])  [unwired: 10 in]
        n154 = case shown="无错误" w403 {
          tunnel: w414 -> [w416 _]
          frame No Error {
            n155 = global write "质控内部交互全局.vi" "氨氮测量状态"(w416) -> ()
            "氨氮测量状态" <- w416
          }
          frame Error {
          }
        }
        n156 = Not(x=w408) -> (.not. x?=w407:bool)
        n157 = global write "质控内部交互全局.vi" "氨氮通讯状态"(w407) -> ()
      }
      frame "总磷读取" {
        n158 = property class="MB_Master"(reference=w420, error in=w419, "Properties:Slave ID"=u8 2 ("Slave ID")) -> (reference out=w423:refnum<class "MB_Master.lvclass">, error out=w429:errorcluster)
        n159 = call <vilib>:"Read Holding Registers.vi"("error in (no error)"=w429, "quantity"=u16 6 ("number of holding registers"), "starting address"=u16 257, "MB session in"=w423) -> ("error out"=w417:errorcluster, "Registers"=w426:u16[], "MB session out"=w418:refnum<class "MB_Master.lvclass">)  [unwired: 5 in]
        n160 = Unbundle By Name(w417) -> ("status"=w422:bool)
        n161 = call "HexToWord.vi"("数组"=w426) -> ("WORD"=w427:u16[])  [unwired: 10 in]
        n162 = case shown="无错误" w417 {
          tunnel: w427 -> [w430 _]
          frame No Error {
            n163 = global write "质控内部交互全局.vi" "总磷测量状态"(w430) -> ()
            "总磷测量状态" <- w430
          }
          frame Error {
          }
        }
        n164 = Not(x=w422) -> (.not. x?=w421:bool)
        n165 = global write "质控内部交互全局.vi" "总磷通讯状态"(w421) -> ()
      }
      frame "总氮读取" {
        n166 = property class="MB_Master"(reference=w434, error in=w433, "Properties:Slave ID"=u8 3 ("Slave ID")) -> (reference out=w441:refnum<class "MB_Master.lvclass">, error out=w435:errorcluster)
        n167 = call <vilib>:"Read Holding Registers.vi"("error in (no error)"=w435, "quantity"=u16 6 ("number of holding registers"), "starting address"=u16 257, "MB session in"=w441) -> ("error out"=w431:errorcluster, "Registers"=w438:u16[], "MB session out"=w432:refnum<class "MB_Master.lvclass">)  [unwired: 5 in]
        n168 = Unbundle By Name(w431) -> ("status"=w442:bool)
        n169 = call "HexToWord.vi"("数组"=w438) -> ("WORD"=w437:u16[])  [unwired: 10 in]
        n170 = case shown="无错误" w431 {
          tunnel: w437 -> [w444 _]
          frame No Error {
            n171 = global write "质控内部交互全局.vi" "总氮测量状态"(w444) -> ()
            "总氮测量状态" <- w444
          }
          frame Error {
          }
        }
        n172 = Not(x=w442) -> (.not. x?=w443:bool)
        n173 = global write "质控内部交互全局.vi" "总氮通讯状态"(w443) -> ()
      }
      frame "CODMn读取" {
        n174 = property class="MB_Master"(reference=w448, error in=w447, "Properties:Slave ID"=u8 4 ("Slave ID")) -> (reference out=w456:refnum<class "MB_Master.lvclass">, error out=w449:errorcluster)
        n175 = call <vilib>:"Read Holding Registers.vi"("error in (no error)"=w449, "quantity"=u16 6 ("number of holding registers"), "starting address"=u16 257, "MB session in"=w456) -> ("error out"=w445:errorcluster, "Registers"=w453:u16[], "MB session out"=w446:refnum<class "MB_Master.lvclass">)  [unwired: 5 in]
        n176 = Unbundle By Name(w445) -> ("status"=w455:bool)
        n177 = call "HexToWord.vi"("数组"=w453) -> ("WORD"=w452:u16[])  [unwired: 10 in]
        n178 = case shown="无错误" w445 {
          tunnel: w452 -> [w458 _]
          frame No Error {
            n179 = global write "质控内部交互全局.vi" "CODMn测量状态"(w458) -> ()
            "CODMn测量状态" <- w458
          }
          frame Error {
          }
        }
        n180 = Not(x=w455) -> (.not. x?=w454:bool)
        n181 = global write "质控内部交互全局.vi" "CODMn通讯状态"(w454) -> ()
      }
      frame "CODCr读取" {
        n182 = property class="MB_Master"(reference=w462, error in=w461, "Properties:Slave ID"=u8 5 ("Slave ID")) -> (reference out=w470:refnum<class "MB_Master.lvclass">, error out=w463:errorcluster)
        n183 = call <vilib>:"Read Holding Registers.vi"("error in (no error)"=w463, "quantity"=u16 6 ("number of holding registers"), "starting address"=u16 257, "MB session in"=w470) -> ("error out"=w459:errorcluster, "Registers"=w467:u16[], "MB session out"=w460:refnum<class "MB_Master.lvclass">)  [unwired: 5 in]
        n184 = Unbundle By Name(w459) -> ("status"=w469:bool)
        n185 = call "HexToWord.vi"("数组"=w467) -> ("WORD"=w466:u16[])  [unwired: 10 in]
        n186 = case shown="无错误" w459 {
          tunnel: w466 -> [w472 _]
          frame No Error {
            n187 = global write "质控内部交互全局.vi" "CODCr测量状态"(w472) -> ()
            "CODCr测量状态" <- w472
          }
          frame Error {
          }
        }
        n188 = Not(x=w469) -> (.not. x?=w468:bool)
        n189 = global write "质控内部交互全局.vi" "CODCr通讯状态"(w468) -> ()
      }
      frame "仪器启动命令" {
        n190 = global read "质控内部交互全局.vi" "仪器启动命令"() -> (w476:T6)
        n191 = Unbundle By Name(w476) -> ("仪器"=w475:enum16{"", "氨氮", "总磷", "总氮", "CODMn", "CODCr"}, "starting address"=w474:u16, "value"=w473:u16)
        n192 = call "单个写入.vi"("Error in"=w477, "value"=w473, "address"=w474, "Slave ID"=w475) -> ("error out"=w479:errorcluster)  [unwired: 7 in]
      }
      frame "多个写入" {
        n193 = global read "质控内部交互全局.vi" "多个写入"() -> (w491:T7)
        n194 = Unbundle By Name(w491) -> ("Slave ID"=w489:u8, "starting address"=w488:u16, "values"=w487:u16[])
        n195 = call "写入参数.vi"("Error in"=w486, "values"=w487, "starting address"=w488, "Slave ID"=w489) -> ("error out"=w480:errorcluster)  [unwired: 7 in]
        n196 = Unbundle By Name(w480) -> ("code"=w485:i32)
        n197 = case shown="错误" w480 {
          tunnel: w485 -> [_ w497]
          tunnel: w484 -> [_ w496]
          tunnel: [0 w495] -> w483
          tunnel: w482 -> [_ w494]
          tunnel: w481 -> [_ w493]
          frame No Error {
          }
          frame Error {
            n198 = case shown="56" w497 {
              tunnel: w494 -> [w499 _]
              tunnel: w493 -> [w498 _]
              tunnel: w496 -> [w502 w510]
              tunnel: [w503 w510] -> w495
              frame 56 {
                n199 = Greater Or Equal?(x=w502, y=3) -> (x >= y?=w500:bool)
                n200 = case shown="假" w500 {
                  tunnel: [w508 0] -> w503
                  tunnel: w502 -> [w507 _]
                  tunnel: w499 -> [w506 _]
                  tunnel: w498 -> [w504 _]
                  frame False {
                    # "重写三次"
                    n201 = Increment(x=w507) -> (x+1=w508:i32)
                    n202 = Enqueue Element(queue=w506, element=cluster{"命令":string} {"命令"="多个写入"} ("元素"), error in (no error)=w504) -> ()  [unwired: 1 in, 3 out]
                  }
                  frame True {
                  }
                }
              }
              frame 1, Default {
                # "其他错误"
              }
            }
          }
        }
      }
      frame "停用模块" {
        n203 = call "质控单元MB_api.vi"("STEP"=enum16{"open", "read", "write", "close"}."close", "Error in"=w513) -> ("error out"=w512:errorcluster, "MB session out"=w511:refnum<class "MB_Master.lvclass">)  [unwired: 7 in, 1 out]
      }
    }
    n204 = Unbundle By Name(w376) -> ("status"=w382:bool, "code"=w372:i32)
    n205 = disable-structure shown="禁用" {
      disable-tunnel: w376 -> [w388 _]
      disable-tunnel: w372 -> [w387 _]
      disable-tunnel: w369 -> [w386 _]
      disable-tunnel: w368 -> [w385 _]
      frame Disabled {
        n206 = case shown="错误" w388 {
          tunnel: w386 -> [_ w391]
          tunnel: w385 -> [_ w390]
          tunnel: w387 -> [_ w389]
          frame No Error {
          }
          frame Error {
            n207 = case shown="1, 默认" w389 {
              tunnel: w391 -> [_ w395]
              tunnel: w390 -> [_ w394]
              frame 56 {
              }
              frame 1, Default {
                n208 = Flush Queue(queue=w395, error in (no error)=w394) -> (queue out=w392:refnum<queue>, error out=w393:errorcluster)  [unwired: 1 out]
                n209 = Enqueue Element(queue=w392, element=cluster{"命令":string} {"命令"="启用模块"} ("元素"), error in (no error)=w393) -> ()  [unwired: 1 in, 3 out]
              }
            }
          }
        }
      }
      frame Enabled {
      }
    }
    n210 = Not(x=w382) -> (.not. x?=→"通讯状态":bool)
  }
  n211 = while "While循环" {
    tunnel: w3 -> [w517]
    tunnel: w8 -> [w516]
    stop <- FALSE stop-if-true
    # "TCP掉线重连"
    n212 = Wait (ms)(milliseconds to wait=u32 10000 ("等待时间（毫秒）")) -> ()  [unwired: 1 out]
    n213 = global read "断电保存全局.vi" "MB通信方式选择"() -> (w515:enum16{"串口", "TCP"})
    n214 = case shown="\"TCP\"" w515 {
      tunnel: w517 -> [_ w522]
      tunnel: w516 -> [_ w521]
      frame "串口", Default {
      }
      frame "TCP" {
        n215 = global read "断电保存全局.vi" "MB session in"() -> (w520:refnum<class "MB_Master.lvclass">)
        n216 = property class="MB_Master"(reference=w520) -> ("Properties:Session Valid"=w523:bool)  [unwired: 1 in, 2 out]
        n217 = case shown="假" w523 {
          tunnel: w522 -> [w525 _]
          tunnel: w521 -> [w524 _]
          frame False {
            n218 = Flush Queue(queue=w525, error in (no error)=w524) -> (queue out=w528:refnum<queue>, error out=w527:errorcluster)  [unwired: 1 out]
            n219 = Enqueue Element(queue=w528, element=cluster{"命令":string} {"命令"="启用模块"} ("元素"), error in (no error)=w527) -> ()  [unwired: 1 in, 3 out]
          }
          frame True {
          }
        }
      }
    }
  }
